vi "checkListed.vi"(0 "Host_Reference":refnum<class "HGF_Reference.lvclass">, 2 "timeout in ms (-1)":i32, 3 "Library":string, 5 "error in (no error)":errorcluster) -> (14 "dup Host_Reference":refnum<class "HGF_Reference.lvclass">, 16 "dup timeout in ms (-1)":i32, 17 "listed?":enum16{"blacklisted", "whitelisted", "unlisted"}(ring), 19 "error out":errorcluster)   [LabVIEW 2009, in "MoAgSy.lvlib" / "MoAgSy_Host.lvclass"]
doc: "<B>public</B> VI compares Library with referenced Hosts blacklist & whitelist.\nReturns blacklisted, whitelisted or unlisted.\n\nF.Berck@gsi.de\nGSI Darmstadt 2009"
uses:
  MoAgSy_Host.lvclass
  HGF_BaseClasses/HGF_Reference/HGF_Reference.lvclass
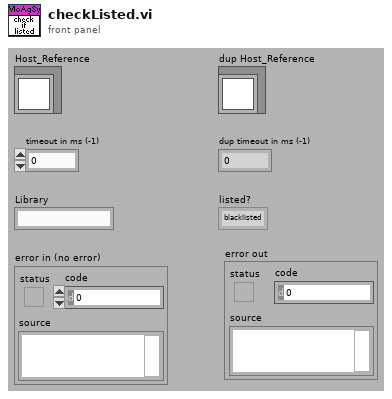
[diagram p1: front panel]
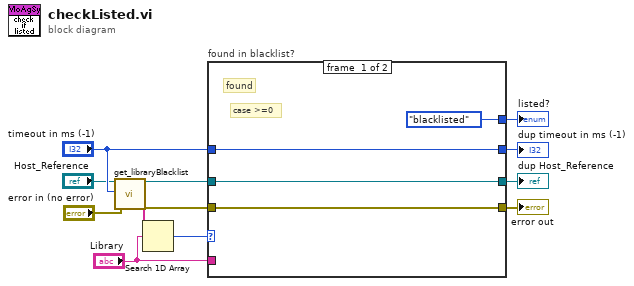
[diagram p0: block diagram]
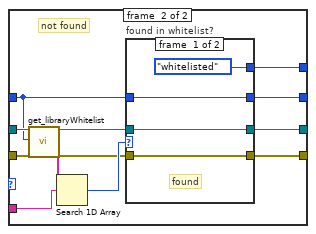
[diagram p2: hidden frame]
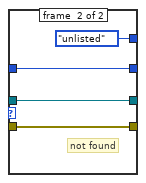
[diagram p3: hidden frame]
diagram:
  n1 = call "get_libraryBlacklist.vi"("Host_Reference"="Host_Reference", "timeout in ms (-1)"="timeout in ms (-1)", "error in (no error)"="error in (no error)") -> ("dup Host_Reference"=w2:refnum<class "HGF_Reference.lvclass">, "Library Blacklist"=w6:string[], "error out"=w5:errorcluster)  [unwired: 14 out]
  n2 = Search 1D Array(1D array=w6, element="Library") -> (index of element=w7:i32)  [unwired: 1 out]
  n3 = case "found in blacklist?" shown="-1" w7 {
    tunnel: w2 -> [w16 w28]
    tunnel: "timeout in ms (-1)" -> [w15 w22]
    tunnel: [w16 w23] -> w12
    tunnel: [w14 w20] -> w1
    tunnel: [w15 w21] -> w10
    tunnel: w5 -> [w14 w18]
    tunnel: "Library" -> [_ w19]
    tunnel: [enum16{"blacklisted", "whitelisted", "unlisted"}."blacklisted" w17] -> w11
    frame #0 {
      # "case >=0"
      # "found"
    }
    frame #1 {
      # "not found"
      n4 = call "get_libraryWhitelist.vi"("Host_Reference"=w28, "timeout in ms (-1)"=w22, "error in (no error)"=w18) -> ("dup Host_Reference"=w25:refnum<class "HGF_Reference.lvclass">, "Library Whitelist"=w27:string[], "error out"=w24:errorcluster)  [unwired: 14 out]
      n5 = Search 1D Array(1D array=w27, element=w19) -> (index of element=w26:i32)  [unwired: 1 out]
      n6 = case "found in whitelist?" shown="0, Default" w26 {
        tunnel: w25 -> [w32 w36]
        tunnel: w24 -> [w30 w34]
        tunnel: [w32 w36] -> w23
        tunnel: w22 -> [w31 w35]
        tunnel: [w31 w35] -> w21
        tunnel: [w30 w34] -> w20
        tunnel: [enum16{"blacklisted", "whitelisted", "unlisted"}."whitelisted" enum16{"blacklisted", "whitelisted", "unlisted"}."unlisted"] -> w17
        frame #0 {
          # "found"
        }
        frame #1 {
          # "not found"
        }
      }
    }
  }
  "dup timeout in ms (-1)" <- w10
  "listed?" <- w11
  "dup Host_Reference" <- w12
  "error out" <- w1
